vi "Lorentzian complex test.vi"(3 "output control":T1, 4 "data":variant, 5 "X":dbl[](array[numeric]), 6 "a":dbl[](array[numeric])) -> (0 "error out":errorcluster, 1 "f'(X,a)":dbl[][](array[numeric]), 2 "f(X,a)":dbl[](array[numeric]))   [LabVIEW 2016]
doc: "Sum of three Gaussians, plus DC offset."
uses:
  <vilib>/gmath/NumericalOptimization/LM_output select.ctl
  <vilib>/gmath/NI_Gmath.lvlib
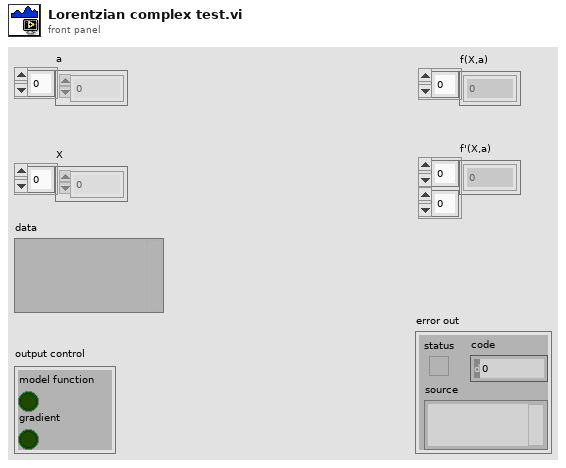
[diagram p1: front panel]
types:
  T1 = typedef "NI_Gmath.lvlib/LM_output select.ctl" = cluster{"model function":bool, "gradient":bool}
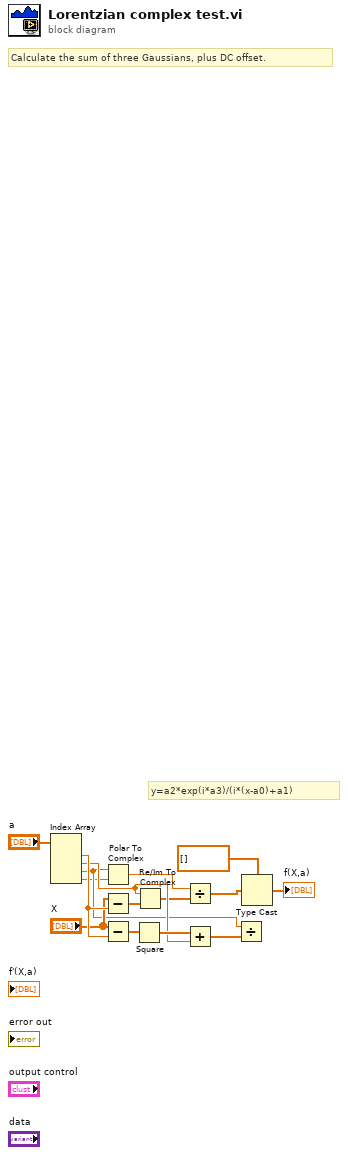
[diagram p0: block diagram]
diagram:
  # "y=a2*exp(i*a3)/(i*(x-a0)+a1)"
  # "Calculate the sum of three Gaussians, plus DC offset."
  n1 = Index Array(array="a") -> (element #1=w10:dbl, element #2=w8:dbl, element #3=w5:dbl, element #4=w4:dbl)  [unwired: 4 in]
  n2 = Polar To Complex(1:w4, 2:w5) -> (0:w7:cdb)
  n3 = Subtract(x="X", y=w10) -> (x-y=w11:dbl[])
  n4 = Subtract(x="X", y=w10) -> (x-y=w14:dbl[])
  n5 = Square(x=w14) -> (x^2=w12:dbl[])
  n6 = Re/Im To Complex(1:w11, 2:w8) -> (0:w6:cdb[])
  n7 = Divide(x=w7, y=w6) -> (x/y=w3:cdb[])
  n8 = Add(x=w12, y=w8) -> (x+y=w13:dbl[])
  n9 = Divide(x=w5, y=w13) -> ()  [unwired: 1 out]
  n10 = Type Cast(type=dbl[] [], x=w3) -> (*(type *) &x=→"f(X,a)":dbl[])
